vi "LCB Write Dev Param.vi"(6 "AdjustEndian":bool, 7 "Data Size":u32, 8 "error in (no error)":errorcluster caption="Fehler (Eingang, kein Fehler)", 9 "Data":u32, 10 "Parameter Identifier":u32, 11 "Device Handle":i64) -> (0 "error out":errorcluster caption="Fehler (Ausgang)")   [LabVIEW 2021, in "labbCAN_Bus_API.lvlib"]
doc: "LCB_Func long __stdcall LCB_WriteDevParam(dev_hdl hDev_in,\n unsigned long DevParamId,\n void *pWriteBuf,\n unsigned long BufSize,\n unsigned char AdjustEndian);"
uses:
  labbCAN_Bus_API.lvlib
  labbCAN_Bus_API.dll
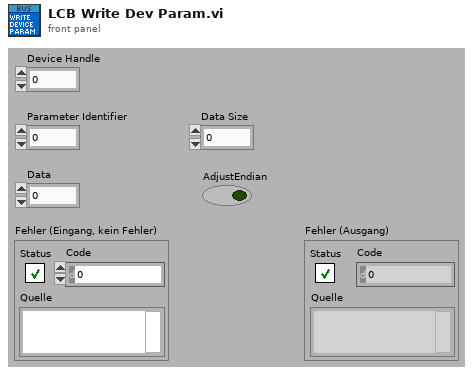
[diagram p1: front panel]
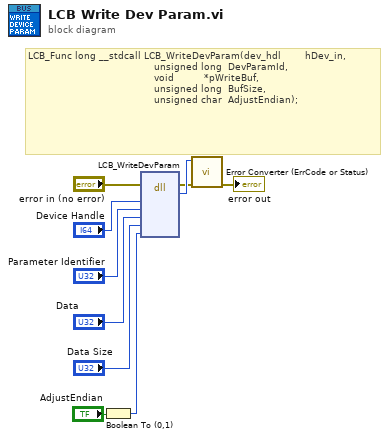
[diagram p0: block diagram]
diagram:
  # "LCB_Func long __stdcall LCB_WriteDevParam(dev_hdl        hDev_in,\n                                          unsigned long  DevParamId,\n                                          void          *pWriteBuf,\n                                          unsigned long  BufSize,\n                                          unsigned char  AdjustEndian);"
  n1 = Boolean To (0,1)(Boolean="AdjustEndian") -> (0, 1=w1:i16)
  n2 = dll-call lib="C:/Users/olaja/AppData/Local/CETONI_SDK/labbCAN_Bus_API.*" fn="LCB_WriteDevParam"(error in="error in (no error)", "hDev_in"="Device Handle", "DevParamId"="Parameter Identifier", "pWriteBuf"="Data", "BufSize"="Data Size", "AdjustEndian"=w1) -> (error out=w4:errorcluster, "Rückgabetyp"=w5:i32)  [unwired: 7 in, 1 out]
  n3 = call "Error Converter (ErrCode or Status).vi"("error in (no error)"=w4, "error code"=w5) -> ("error out"=→"error out":errorcluster)  [unwired: 9 in]
